vi "Read Gauge Activation Configuration.vi"(7 "gauge":u16(ring)=1 items=["1"=1, "2"=2, "3"=3], 8 "error in (no error)":errorcluster, 11 "VGC in":refnum<class "PL Inficon VGC.lvclass">) -> (0 "error out":errorcluster, 1 "deactivation":u16(ring) items=["manual"=0, "self control"=1, "channel 1"=3, "channel 2"=4, "channel 3"=5], 2 "activation":u16(ring) items=["manual"=0, "hot start"=1, "channel 1"=3, "channel 2"=4, "channel 3"=5], 3 "VGC out":refnum<class "PL Inficon VGC.lvclass">, 4 "thresholds":cluster{"on":dbl, "off":dbl})   [LabVIEW 2015, in "PL Inficon VGC.lvclass"]
doc: "Reads gauge activation configuration."
uses:
  PL Inficon VGC.lvclass
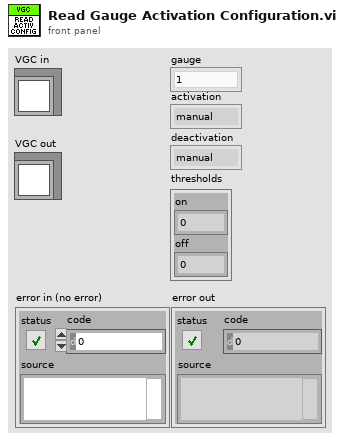
[diagram p1: front panel]
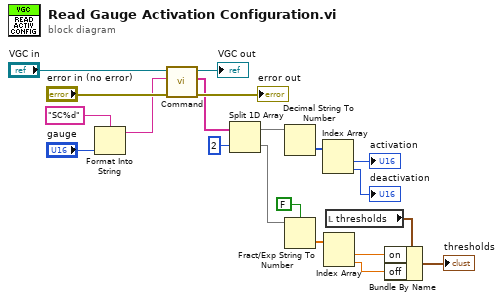
[diagram p0: block diagram]
diagram:
  n1 = Format Into String(format string="SC%d", "gauge") -> (resulting string=w8:string)  [unwired: 2 in, 1 out]
  n2 = call "Command.vi"("error in (no error)"="error in (no error)", "command"=w8, "VGC in"="VGC in") -> ("error out"=→"error out":errorcluster, "response data"=w15:string[], "VGC out"=→"VGC out":refnum<class "PL Inficon VGC.lvclass">)  [unwired: 6 in]
  n3 = Split 1D Array(array=w15, index=2) -> (first subarray=w13:string[], second subarray=w12:string[])
  n4 = Decimal String To Number(string=w13) -> (number=w7:i32[])  [unwired: 2 in, 1 out]
  n5 = Fract/Exp String To Number(use system decimal point (T)=FALSE, string=w12) -> (number=w11:dbl[])  [unwired: 2 in, 1 out]
  n6 = Index Array(array=w7) -> (element #1=→"activation":i32, element #2=→"deactivation":i32)  [unwired: 2 in]
  n7 = Index Array(array=w11) -> (element #1=w3:dbl, element #2=w2:dbl)  [unwired: 2 in]
  n8 = local read "thresholds"() -> (w4:cluster{"on":dbl, "off":dbl})
  n9 = Bundle By Name(cluster=w4, "on"=w3, "off"=w2) -> (→"thresholds":cluster{"on":dbl, "off":dbl})
